vi "main.vi"() -> ()   [LabVIEW 2018]
panel:
  out "substring 2":string
  out "substring":string
  out "error out 16":errorcluster
  out "error out 15":errorcluster
  out "error out 14":errorcluster
  out "error out 13":errorcluster
  out "error out 12":errorcluster
  out "error out 11":errorcluster
  out "error out 10":errorcluster
  out "error out 9":errorcluster
  out "error out 8":errorcluster
  out "error out 7":errorcluster
  out "error out 6":errorcluster
  out "error out 5":errorcluster
  out "error out 4":errorcluster
  out "error out 3":errorcluster
  out "Boolean":bool
  out "Password":string="tetris"
  out "Board 2":picture
  in  "Array 3":dbl[][](array[numeric])
  out "Array":i32[][](array[numeric])
  in  "?":u16(ring) items=["Single Player", "Double Player"]
  out "Next Piece":picture
  out "Score":u32
  out "Rows Cleared":u16
  in  "Difficulty":u16(ring) items=["Easy", "Medium", "Hard"]
  out "Board":picture
  out "error out 2":errorcluster
  out "error out":errorcluster
  in  "?":bool
  out "wait mS":u16=250
  # "CHIRSTMAST EDITION !!!"
  # "TETRIS"
  # "LET'S PLAY !!!"
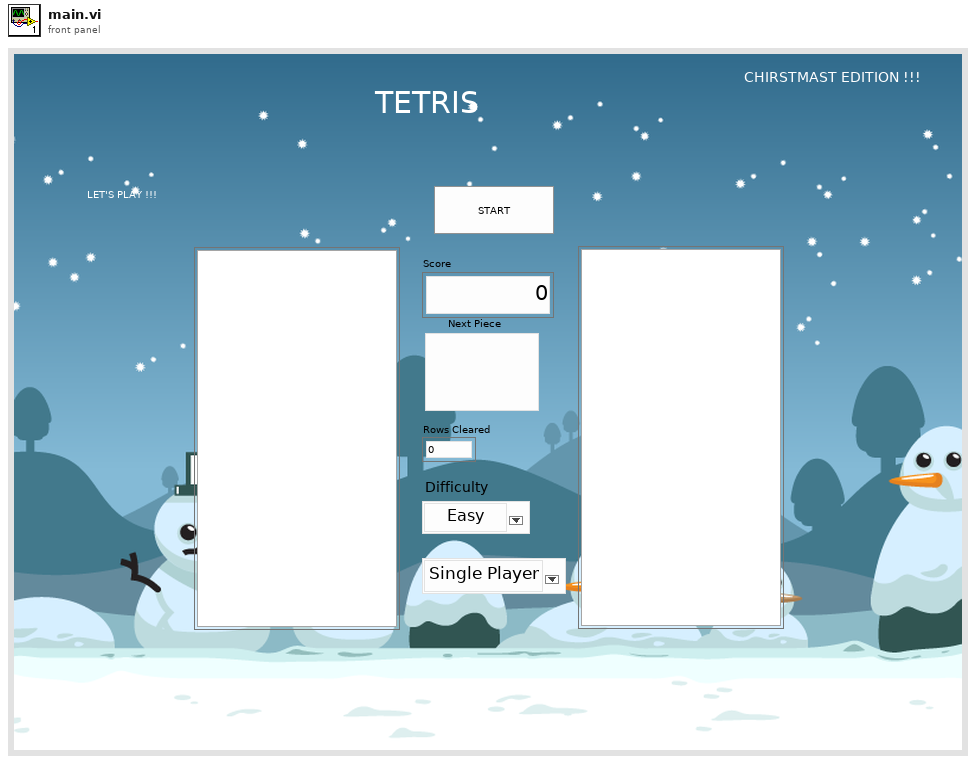
[diagram p1: front panel]
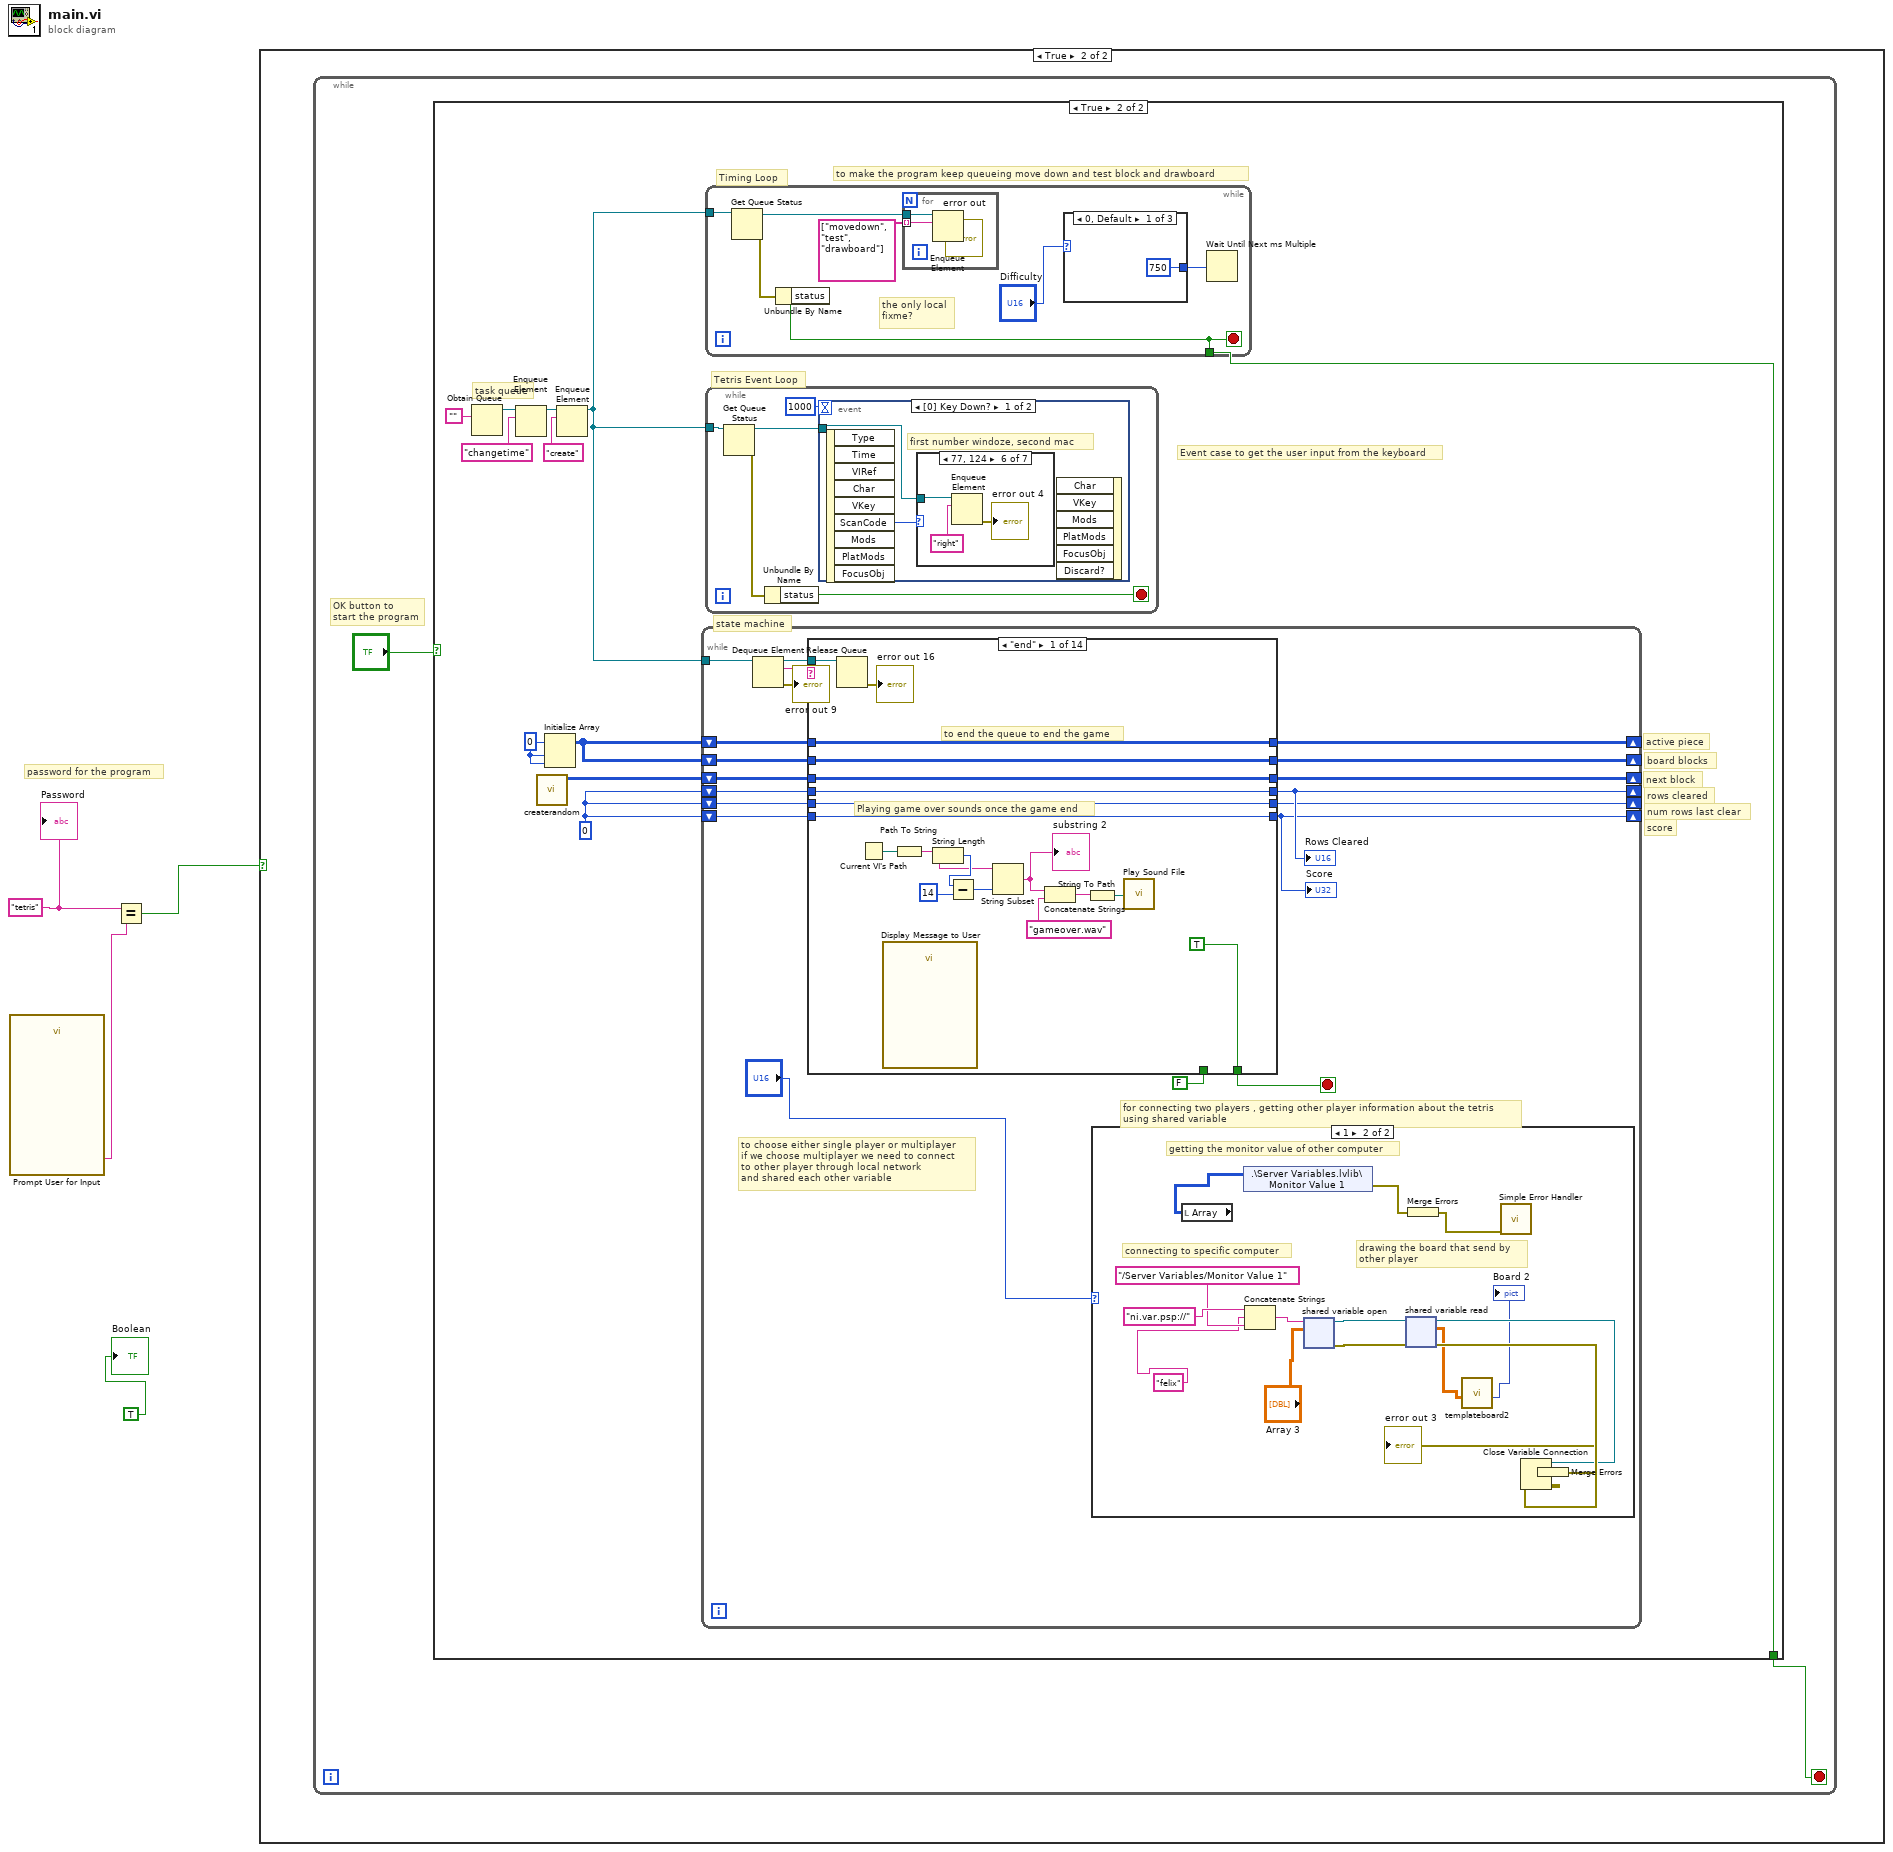
[diagram p0: block diagram]
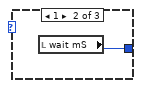
[diagram p4: hidden frame]
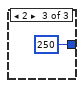
[diagram p5: hidden frame]
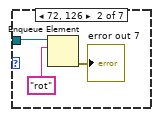
[diagram p7: hidden frame]
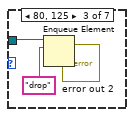
[diagram p8: hidden frame]
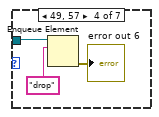
[diagram p9: hidden frame]
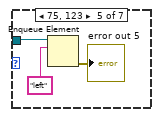
[diagram p10: hidden frame]
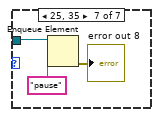
[diagram p11: hidden frame]
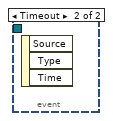
[diagram p12: hidden frame]
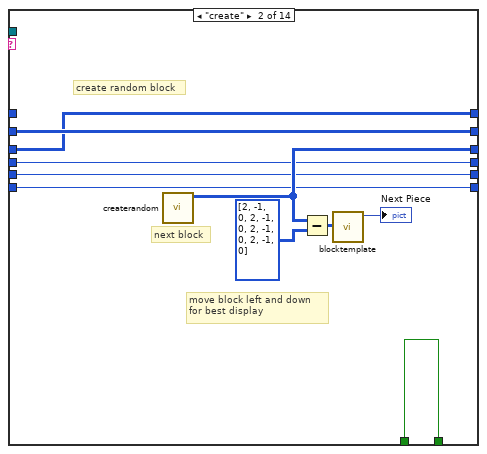
[diagram p14: hidden frame]
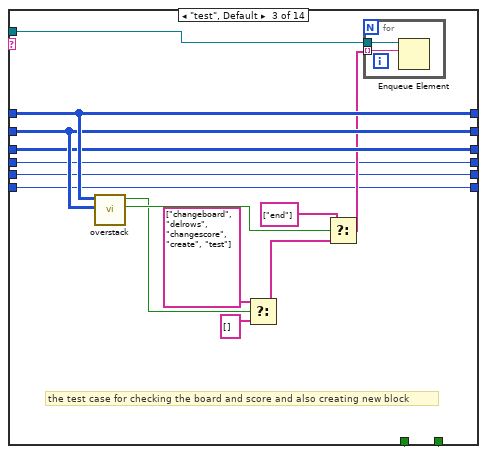
[diagram p15: hidden frame]
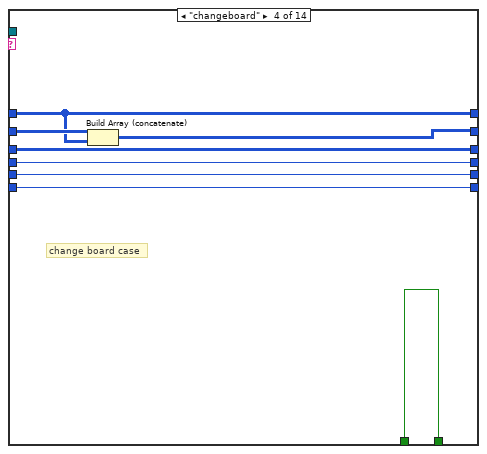
[diagram p16: hidden frame]
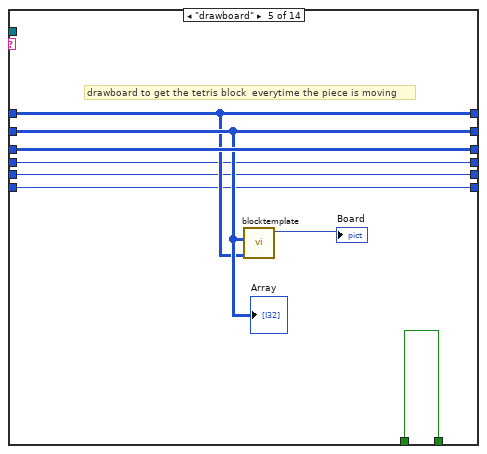
[diagram p17: hidden frame]
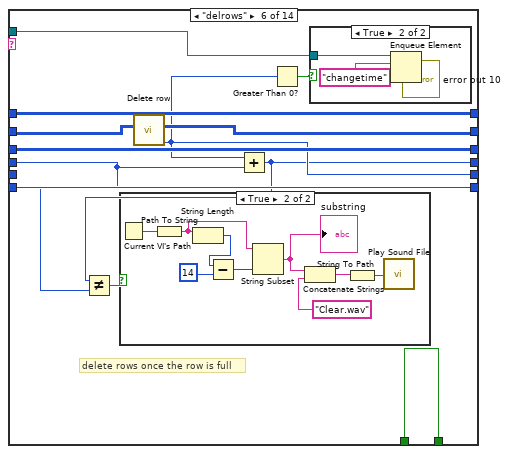
[diagram p18: hidden frame]
diagram:
  w3 = "tetris" ("String")
  # "password for the program"
  n1 = call "Prompt User for Input"() -> ("Input password"=w4:string)  [unwired: 17 in, 2 out]
  n2 = Equal?(x=w3, y=w4) -> (x = y?=w2:bool)
  n3 = case shown="True" w2 {
    frame False {
    }
    frame True {
      n4 = while {
        stop <- w5 stop-if-true
        # "OK button to \nstart the program"
        n5 = case shown="True" "?" {
          tunnel: [_ w7] -> w5
          frame False {
          }
          frame True {
            w8 = 0
            w16 = 0
            # "Event case to get the user input from the keyboard"
            # "to make the program keep queueing move down and test block and drawboard"
            # "task queue"
            # "num rows last clear"
            # "score"
            # "rows cleared"
            # "Timing Loop"
            # "Tetris Event Loop"
            # "state machine"
            # "next block"
            # "board blocks"
            # "active piece"
            n6 = Obtain Queue(element data type="") -> (queue out=w14:refnum<queue>)  [unwired: 4 in, 2 out]
            n7 = Enqueue Element(queue=w14, element="changetime") -> (queue out=w11:refnum<queue>)  [unwired: 2 in, 2 out]
            n8 = call "createrandom.vi"() -> ("Array"=w17:i32[][])  [unwired: 11 in]
            n9 = Initialize Array(w16, w16, w16) -> (w12:i32[][])
            n10 = Enqueue Element(queue=w11, element="create") -> (queue out=w10:refnum<queue>)  [unwired: 2 in, 2 out]
            n11 = while {
              shift-right: [w64] -> _
              shift-left: w12 -> [w72]
              shift-right: [w65] -> _
              shift-left: w12 -> [w71]
              shift-right: [w69] -> _
              shift-left: w17 -> [w70]
              tunnel: w10 -> [w68]
              shift-right: [w62] -> _
              shift-left: w8 -> [w63]
              shift-right: [w59] -> _
              shift-left: w8 -> [w60]
              shift-right: [w58] -> _
              shift-left: w8 -> [w61]
              stop <- w73 stop-if-true
              # "to choose either single player or multiplayer\nif we choose multiplayer we need to connect \nto other player through local network \nand shared each other variable"
              # "for connecting two players , getting other player information about the tetris\nusing shared variable"
              n12 = Dequeue Element(queue=w68) -> (queue out=w67:refnum<queue>, element=w66:string, error out=→"error out 9":errorcluster)  [unwired: 2 in, 1 out]
              n13 = case shown="\"end\"" w66 {
                tunnel: FALSE -> [_ w109 w133 w143 w151 w163 w190 w202 w209 w220 w242 w257 w269 w282]
                tunnel: [TRUE w109 w133 w143 w151 w163 w190 w202 w209 w220 w242 w257 w269 w282] -> w73
                tunnel: [w107 w117 w132 w141 w148 w162 w189 w204 w210 w218 w236 w249 w266 w280] -> w64
                tunnel: w72 -> [w107 _ w132 w141 w148 w162 w189 w204 w212 w218 w237 w251 w267 w280]
                tunnel: w71 -> [w106 w118 w131 w142 w149 w161 w187 w203 w213 w221 w235 w250 w265 w279]
                tunnel: [w106 w118 w131 w140 w149 w160 w187 w203 w213 w221 w235 w250 w265 w279] -> w65
                tunnel: w70 -> [w105 w117 w127 w139 w150 w159 w188 w201 w208 w219 w241 w256 w268 w281]
                tunnel: [w105 w116 w127 w139 w150 w159 w188 w201 w208 w219 w241 w256 w268 w281] -> w69
                tunnel: w67 -> [w101 _ w126 _ _ w158 _ _ _ w217 w232 w247 w258 w276]
                tunnel: [w104 w112 w121 w138 w146 w154 w185 w198 w207 w216 w240 w255 w264 w274] -> w62
                tunnel: w63 -> [w104 w112 w121 w138 w146 w153 w185 w198 w207 w216 w240 w255 w264 w274]
                tunnel: [w103 w111 w120 w137 w145 w155 w184 w196 w206 w215 w239 w254 w263 w273] -> w59
                tunnel: [w102 w110 w119 w136 w144 w157 w186 w192 w205 w214 w238 w253 w262 w272] -> w58
                tunnel: w61 -> [w102 w110 w119 w136 w144 w157 w186 w200 w205 w214 w238 w253 w262 w272]
                tunnel: w60 -> [w103 w111 w120 w137 w145 _ w184 w196 w206 w215 w239 w254 w263 w273]
                frame "end" {
                  # "to end the queue to end the game"
                  # "Playing game over sounds once the game end"
                  n14 = Release Queue(queue=w101) -> (error out=→"error out 16":errorcluster)  [unwired: 2 in, 2 out]
                  n15 = Current VI's Path() -> (path=w98:path)
                  n16 = call "Display Message to User"() -> ()  [unwired: 10 in, 2 out]
                  n17 = Path To String(path=w98) -> (string=w91:string)
                  n18 = String Length(string=w91) -> (length=w95:i32)
                  n19 = Subtract(x=w95, y=14) -> (x-y=w93:i32)
                  n20 = String Subset(string=w91, length (rest)=w93) -> (substring=w92:string)  [unwired: 1 in]
                  "substring 2" <- w92
                  n21 = Concatenate Strings(w92, "gameover.wav" ("string")) -> (w99:string)
                  n22 = String To Path(string=w99) -> (path=w97:path)
                  n23 = call <vilib>:"Play Sound File.vi"("path"=w97) -> ()  [unwired: 9 in, 2 out]
                }
                frame "create" {
                  # "create random block"
                  # "move block left and down\nfor best display"
                  # "next block"
                  n24 = call "createrandom.vi"() -> ("Array"=w116:i32[][])  [unwired: 11 in]
                  n25 = Subtract(x=w116, y=i32[][] [[2, -1, 0], [2, -1, 0], [2, -1, 0], [2, -1, 0]]) -> (x-y=w114:i32[][])
                  n26 = call "blocktemplate.vi"("Piece Array"=w114) -> ("Picture"=→"Next Piece":picture)  [unwired: 10 in]
                }
                frame "test", Default {
                  # "the test case for checking the board and score and also creating new block"
                  n27 = call "overstack.vi"("board array"=w131, "Piece Array"=w132) -> ("Lost"=w129:bool, "Touching"=w128:bool)  [unwired: 7 in, 1 out]
                  n28 = Select(t=string[] ["changeboard", "delrows", "changescore", "create", "test"], s=w128, f=string[] []) -> (s? t:f=w130:string[])
                  n29 = Select(t=string[] ["end"], s=w129, f=w130) -> (s? t:f=w125:string[])
                  n30 = for {
                    tunnel: w126 -> [w135]
                    tunnel: w125 -> [w134] mode=indexing
                    n31 = Enqueue Element(queue=w135, element=w134) -> ()  [unwired: 2 in, 3 out]
                  }
                }
                frame "changeboard" {
                  # "change board case"
                  n32 = Build Array (concatenate)(w142, w141) -> (w140:i32[][])
                }
                frame "drawboard" {
                  # "drawboard to get the tetris block  everytime the piece is moving"
                  n33 = call "blocktemplate.vi"("Piece Array"=w148, "board array"=w149) -> ("Picture"=→"Board":picture)  [unwired: 9 in]
                  "Array" <- w149
                }
                frame "delrows" {
                  # "delete rows once the row is full"
                  n34 = call "Delete row.vi"("tetris block"=w161) -> ("Rows Deleted"=w155:u16, "new tetris block"=w160:u8[][])  [unwired: 9 in]
                  n35 = Add(x=w155, y=w153) -> (x+y=w154:i32)
                  n36 = Not Equal?(x=w154, y=w153) -> (x != y?=w152:bool)
                  n37 = case shown="True" w152 {
                    frame False {
                    }
                    frame True {
                      n38 = Current VI's Path() -> (path=w171:path)
                      n39 = Path To String(path=w171) -> (string=w165:string)
                      n40 = String Length(string=w165) -> (length=w168:i32)
                      n41 = Subtract(x=w168, y=14) -> (x-y=w166:i32)
                      n42 = String Subset(string=w165, length (rest)=w166) -> (substring=w164:string)  [unwired: 1 in]
                      "substring" <- w164
                      n43 = Concatenate Strings(w164, "Clear.wav" ("string")) -> (w172:string)
                      n44 = String To Path(string=w172) -> (path=w170:path)
                      n45 = call <vilib>:"Play Sound File.vi"("path"=w170) -> ()  [unwired: 9 in, 2 out]
                    }
                  }
                  n46 = Greater Than 0?(x=w155) -> (x > 0?=w156:bool)
                  n47 = case shown="True" w156 {
                    tunnel: w158 -> [_ w174]
                    frame False {
                    }
                    frame True {
                      n48 = Enqueue Element(queue=w174, element="changetime") -> (error out=→"error out 10":errorcluster)  [unwired: 2 in, 2 out]
                    }
                  }
                }
                frame "changetime" {
                  w179 = 100
                  w182 = 10
                  # "start time"
                  # "wait time the only local in this example"
                  n49 = Quotient & Remainder(x=w185, y=w182) -> (floor(x/y)=w183:i32)  [unwired: 1 out]
                  n50 = Multiply(x=w183, y=w182) -> (x*y=w181:i32)
                  n51 = Subtract(x=w179, y=w181) -> (x-y=w180:i32)
                  n52 = Divide(x=w180, y=w179) -> (x/y=w178:dbl)
                  n53 = Multiply(x=w178, y=500) -> (x*y=→"wait mS":dbl)
                }
                frame "changescore" {
                  # "the score calculation , the more row clear at once \nthe higher the score we get at once"
                  n54 = Index Array(array=i32[] [1, 40, 100, 300, 1200], index=w196) -> (element=w193:i32)
                  n55 = Quotient & Remainder(x=w198, y=10) -> (floor(x/y)=w197:i32)  [unwired: 1 out]
                  n56 = Increment(x=w197) -> (x+1=w194:i32)
                  n57 = Multiply(x=w194, y=w193) -> (x*y=w191:i32)
                  n58 = Add(x=w200, y=w191) -> (x+y=w192:i32)
                }
                frame "movedown" {
                  # "moving down the tetris piece"
                  n59 = Add(x=w212, y=i32[][] [[0, 1, 0], [0, 1, 0], [0, 1, 0], [0, 1, 0]]) -> (x+y=w210:i32[][])
                }
                frame "pause" {
                  # "to pause the game"
                  # "pop values off the stack\nchecking for \"pause\""
                  n60 = while {
                    tunnel: w217 -> [w227]
                    stop <- w224 stop-if-true
                    n61 = Dequeue Element(queue=w227) -> (element=w225:string, error out=→"error out 11":errorcluster)  [unwired: 2 in, 2 out]
                    n62 = Wait (ms)(milliseconds to wait=25) -> ()  [unwired: 1 out]
                    n63 = Equal?(x=w225, y="pause") -> (x = y?=w224:bool)
                  }
                }
                frame "right" {
                  # "to move right the piece"
                  n64 = Enqueue Element(queue=w232, element="test") -> (queue out=w230:refnum<queue>, error out=→"error out 15":errorcluster)  [unwired: 2 in, 1 out]
                  n65 = Enqueue Element(queue=w230, element="drawboard") -> (error out=→"error out 14":errorcluster)  [unwired: 2 in, 2 out]
                  n66 = call "Shift left right.vi"("TETRIS BLOCK"=w237, "Filled Array"=w235, "Move Right"=TRUE) -> ("After Shift"=w236:u8[][])  [unwired: 6 in]
                }
                frame "left" {
                  # "to move the piece to the left"
                  n67 = Enqueue Element(queue=w247, element="test") -> (queue out=w246:refnum<queue>, error out=→"error out 12":errorcluster)  [unwired: 2 in, 1 out]
                  n68 = Enqueue Element(queue=w246, element="drawboard") -> (error out=→"error out 13":errorcluster)  [unwired: 2 in, 2 out]
                  n69 = call "Shift left right.vi"("TETRIS BLOCK"=w251, "Filled Array"=w250, "Move Right"=FALSE) -> ("After Shift"=w249:u8[][])  [unwired: 6 in]
                }
                frame "rot" {
                  # "to rotate the piece that are falling\nand drawbaord everytime it changes"
                  n70 = Enqueue Element(queue=w258, element="test") -> (queue out=w260:refnum<queue>)  [unwired: 2 in, 2 out]
                  n71 = Enqueue Element(queue=w260, element="drawboard") -> ()  [unwired: 2 in, 3 out]
                  n72 = call "rotate.vi"(9:w265, 11:w267) -> (3:w266:u8[][])  [unwired: 9 in]
                }
                frame "drop" {
                  # "to drop the piece we use movedown repetatedly until\nthe piece touch the stack"
                  n73 = call "overstack.vi"("board array"=w279, "Piece Array"=w280) -> ("min Distance"=w271:i16)  [unwired: 7 in, 2 out]
                  n74 = Decrement(x=w271) -> (x-1=w270:i16)
                  n75 = for {
                    N: w270 -> [_]
                    tunnel: ["movedown"] -> w278 mode=indexing
                  }
                  n76 = Build Array (concatenate)(w278, "test") -> (w275:string[])
                  n77 = for {
                    tunnel: w276 -> [w284]
                    tunnel: w275 -> [w283] mode=indexing
                    n78 = Enqueue Element(queue=w284, element=w283) -> ()  [unwired: 2 in, 3 out]
                  }
                }
              }
              "Rows Cleared" <- w62
              "Score" <- w58
              n79 = case shown="1" "?" {
                frame 0, Default {
                }
                frame 1 {
                  # "drawing the board that send by \nother player"
                  # "connecting to specific computer"
                  # "getting the monitor value of other computer"
                  n80 = local read "Array"() -> (w81:i32[][])
                  n81 = shared-variable ".\\Server Variables.lvlib\\Monitor Value 1"(w81) -> (error out=w85:errorcluster)  [unwired: 1 in]
                  n82 = Concatenate Strings("ni.var.psp://" ("string"), "felix", "/Server Variables/Monitor Value 1") -> (w88:string)
                  n83 = shared-variable-open(w88, "Array 3") -> (w90:refnum<k21>, w89:errorcluster)  [unwired: 2 in]
                  n84 = shared-variable-read(w90, w89) -> (w83:refnum<k21>, w84:errorcluster, w75:dbl[][])  [unwired: 1 out]
                  n85 = Merge Errors(w85) -> (w86:errorcluster)
                  n86 = call "templateboard2.vi"("board array"=w75) -> ("Picture"=→"Board 2":picture)  [unwired: 10 in]
                  n87 = call <vilib>:"Simple Error Handler.vi"("error in (no error)"=w86) -> ()  [unwired: 4 in, 5 out]
                  n88 = Close Variable Connection(8:w84, 11:w83) -> (0:w82:errorcluster)
                  n89 = Merge Errors(w82) -> (→"error out 3":errorcluster)
                }
              }
            }
            n90 = while {
              tunnel: w10 -> [w22]
              tunnel: [w18] -> w7
              stop <- w18 stop-if-true
              # "the only local\nfixme?"
              n91 = Get Queue Status(queue=w22) -> (queue out=w21:refnum<queue>, error out=w23:errorcluster)  [unwired: 2 in, 6 out]
              n92 = Unbundle By Name(w23) -> ("status"=w18:bool)
              n93 = for {
                tunnel: w21 -> [w30]
                tunnel: string[] ["movedown", "test", "drawboard"] -> [w29] mode=indexing
                n94 = Enqueue Element(queue=w30, element=w29) -> (error out=→"error out":errorcluster)  [unwired: 2 in, 2 out]
              }
              n95 = case shown="0, Default" "Difficulty" {
                tunnel: [u16 750 ("wait mS") w26 u16 250 ("wait mS")] -> w20
                frame 0, Default {
                }
                frame 1 {
                  n96 = local read "wait mS"() -> (w26:u16)
                }
                frame 2 {
                }
              }
              n97 = Wait Until Next ms Multiple(millisecond multiple=w20) -> ()  [unwired: 1 out]
            }
            n98 = while {
              tunnel: w10 -> [w32]
              stop <- w33 stop-if-true
              n99 = Get Queue Status(queue=w32) -> (queue out=w31:refnum<queue>, error out=w34:errorcluster)  [unwired: 2 in, 6 out]
              n100 = Unbundle By Name(w34) -> ("status"=w33:bool)
              n101 = event shown="[0] Key Down?" {
                selector: _ -> [_ _]
                dyn-events: _ -> [_ _]
                timeout: 1000 -> [_ _]
                tunnel: w31 -> [w36 _]
                event Key Down? {
                  # "first number windoze, second mac"
                  n102 = event-data() -> ("ScanCode"=w37:i16)  [unwired: 1 in, 8 out]
                  n103 = case shown="77, 124" w37 {
                    tunnel: w36 -> [_ w40 w43 w46 w49 w52 w55]
                    frame 0, Default {
                    }
                    frame 72, 126 {
                      n104 = Enqueue Element(queue=w40, element="rot") -> (error out=→"error out 7":errorcluster)  [unwired: 2 in, 2 out]
                    }
                    frame 80, 125 {
                      n105 = Enqueue Element(queue=w43, element="drop") -> (error out=→"error out 2":errorcluster)  [unwired: 2 in, 2 out]
                    }
                    frame 49, 57 {
                      n106 = Enqueue Element(queue=w46, element="drop") -> (error out=→"error out 6":errorcluster)  [unwired: 2 in, 2 out]
                    }
                    frame 75, 123 {
                      n107 = Enqueue Element(queue=w49, element="left") -> (error out=→"error out 5":errorcluster)  [unwired: 2 in, 2 out]
                    }
                    frame 77, 124 {
                      n108 = Enqueue Element(queue=w52, element="right") -> (error out=→"error out 4":errorcluster)  [unwired: 2 in, 2 out]
                    }
                    frame 25, 35 {
                      n109 = Enqueue Element(queue=w55, element="pause") -> (error out=→"error out 8":errorcluster)  [unwired: 2 in, 2 out]
                    }
                  }
                  n110 = event-data() -> ()  [unwired: 7 in, 1 out]
                }
                event Timeout {
                  n111 = event-data() -> ()  [unwired: 1 in, 3 out]
                }
              }
            }
          }
        }
      }
    }
  }
  "Password" <- w3
  "Boolean" <- TRUE
